vi "Perform Action.vi"(8 "error in":errorcluster, 10 "Input":variant, 11 "AI DAQmx Cont CFG Simulated in":refnum<class "AI DAQmx Cont CFG Simulated.lvclass">) -> (0 "error out":errorcluster, 2 "Output":variant, 3 "AI DAQmx Cont CFG Simulated out":refnum<class "AI DAQmx Cont CFG Simulated.lvclass">)   [LabVIEW 2023, in "DAQmx Simulated CFGs.lvlib" / "AI DAQmx Cont CFG Simulated.lvclass"]
uses:
  AI DAQmx Cont CFG Simulated.lvclass
  AI Cont CFG/AI DAQmx Cont CFG.lvclass/AI DAQmx Cont CFG.ctl
  Configuration/Configuration JSON/Configuration JSON Base/CFG JSON.lvclass/CFG JSON.ctl
  9e247467-b14e-496b-b9e3-e1b64cc5dba4.vi
  <vilib>/JDP Science/JSONtext/Find Item.vi
  <vilib>/JDP Science/JSONtext/Next JSON Value.vi
  <vilib>/JDP Science/JSONtext/String Subset.vi
  <vilib>/JDP Science/JSONtext/Parsing/Advance past next JSON Value (inlined COPY).vi
  <vilib>/JDP Science/JSONtext/Parsing/Advance past whitespace.vi
  <vilib>/JDP Science/JSONtext/Parsing/Advance past String.vi
  <vilib>/JDP Science/JSONtext/Parsing/Advance past Number.vi
  <vilib>/JDP Science/JSONtext/Parsing/Advance past Line Ending.vi
  <vilib>/JDP Science/JSONtext/Parsing/Parse Full Path or Item Name.vi
  <vilib>/JDP Science/JSONtext/Parsing/Advance past Array.vi
  <vilib>/JDP Science/JSONtext/Parsing/Advance past Object.vi
  <vilib>/JDP Science/JSONtext/support/Error Cluster From Code.vi
  <vilib>/JDP Science/JSONtext/Offset/Find Item Locations by Path.vi
  <vilib>/JDP Science/JSONtext/JSON text to Variant.vi
  DAQmx/BufferLastReadingsDBL/BufferLastReadings DBL.lvclass
  <vilib>/JDP Science/JSONtext/LVClass Serializer/JSONtext LVClass Serializer.lvclass
  AI DAQmx Cont CFG Simulated.lvclass/AI DAQmx Cont CFG Simulated.ctl
  Configuration/Configuration JSON/Configuration JSON Base/CFG JSON.lvclass
  AI Cont CFG/AI DAQmx Cont CFG.lvclass
  D:/git/HAL/HAL GOOP4/AI/AI Cont CFG/AI DAQmx Cont CFG.lvclass
  D:/git/HAL/HAL GOOP4/DAQmx/DAQmx Base CFG/DAQmx Base CFG.lvclass
  D:/git/HAL/HAL GOOP4/CFG Target/CFG Target.lvclass
  D:/git/HAL/HAL GOOP4/Configuration/Configuration Semaphore/CFG Semaphore.lvclass
  D:/git/HAL/HAL GOOP4/Configuration/Configuration JSON/Configuration JSON Base/CFG JSON.lvclass
  D:/git/HAL/HAL GOOP4/Interfaces/IConfigure/IConfigure.lvclass
  D:/git/HAL/HAL GOOP4/AI/AI Simulated CFGs/AI DAQmx Cont CFG Simulated.lvclass
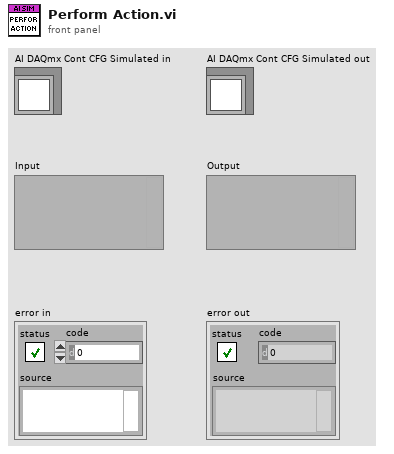
[diagram p1: front panel]
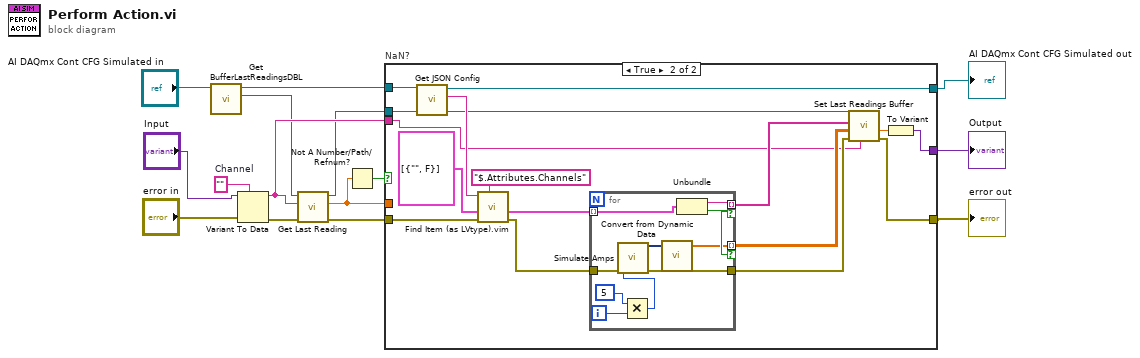
[diagram p0: block diagram]
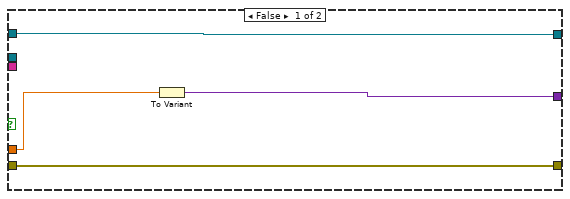
[diagram p2: hidden frame]
diagram:
  w10 = ""  # Channel
  n1 = call "Get BufferLastReadingsDBL.vi"("AI DAQmx Cont CFG in"="AI DAQmx Cont CFG Simulated in") -> ("BufferLastReadings DBL"=w7:refnum<class "BufferLastReadings DBL.lvclass">, "AI DAQmx Cont CFG out"=w6:refnum<class "AI DAQmx Cont CFG Simulated.lvclass">)  [unwired: 9 in]
  n2 = Variant To Data(error in="error in", type=w10, Variant="Input") -> (data=w11:string, error out=w15:errorcluster)
  n3 = call-dynamic "Get Last Reading.vi"("error in"=w15, "Channel"=w11, "BufferLastReadingsDBL in"=w7) -> ("error out"=w13:errorcluster, "Reading"=w12:dbl, "BufferLastReadingsDBL out"=w5:refnum<class "BufferLastReadings DBL.lvclass">)  [unwired: 6 in]
  n4 = Not A Number/Path/Refnum?(number/path/refnum=w12) -> (NaN/Path/Refnum?=w14:bool)
  n5 = case "NaN?" shown="True" w14 {
    tunnel: w6 -> [w17 w35]
    tunnel: w13 -> [w16 w33]
    tunnel: [w16 w23] -> w1
    tunnel: [w18 w21] -> w4
    tunnel: [w17 w28] -> w2
    tunnel: w12 -> [w19 _]
    tunnel: w11 -> [_ w20]
    tunnel: w5 -> [_ w27]
    frame False {
      n6 = To Variant(anything=w19) -> (Variant=w18:variant)
    }
    frame True {
      n7 = call "Get JSON Config.vi"("CFG Base in"=w35) -> ("<JSON>Config>"=w34:string, "CFG Base out"=w28:refnum<class "AI DAQmx Cont CFG Simulated.lvclass">)  [unwired: 9 in]
      n8 = call "Find Item (as LVtype).vim"("$Path or Item Name"="$.Attributes.Channels", "error in (no error)"=w33, "Data Type and Default Value"=cluster{"Name":string, "Enabled":bool}[] [{"Name"="", "Enabled"=FALSE}], "JSON"=w34) -> ("error out"=w29:errorcluster, "Data"=w30:cluster{"Name":string, "Enabled":bool}[])  [unwired: 4 in, 2 out]
      n9 = for {
        tunnel: w30 -> [w45] mode=indexing
        tunnel: [w44] -> w26 mode=indexing if=w41
        tunnel: w29 -> [w43]
        tunnel: [w42] -> w24
        tunnel: [w36] -> w25 mode=indexing if=w41
        i -> [w40]
        n10 = Multiply(x=5, y=w40) -> (x*y=w38:i32)
        n11 = call "Simulate Amps"("Phase"=w38, "error in (no error)"=w43) -> ("Sine Amps 0.0015"=w37:dynamicdata, "error out"=w42:errorcluster)  [unwired: 12 in]
        n12 = call "Convert from Dynamic Data"("Dynamic Data Type"=w37) -> ("Array"=w36:dbl[])  [unwired: 3 in]
        n13 = Unbundle(w45) -> ("Name"=w44:string, "Enabled"=w41:bool)
      }
      n14 = call-dynamic "Set Last Readings Buffer.vi"("Read Channel Ident"=w20, "error in"=w24, "Readings"=w25, "Channel Idents"=w26, "BufferLastReadingsDBL in"=w27) -> ("error out"=w23:errorcluster, "Reading"=w22:dbl)  [unwired: 4 in, 1 out]
      n15 = To Variant(anything=w22) -> (Variant=w21:variant)
    }
  }
  "error out" <- w1
  "AI DAQmx Cont CFG Simulated out" <- w2
  "Output" <- w4
